vi "Build Chart Update.vi"(4 "error in (no error)":errorcluster, 7 "State Machine Data":T2) -> (0 "error out":errorcluster, 3 "Chart Sample":T1)   [LabVIEW 2015, in "Startup Processes.lvlib"]
uses:
  Startup Processes.lvlib
  _typedefs/State Machine Conditions.ctl
  _typedefs/Machine Modes.ctl
  _typedefs/Subpanel Names.ctl
  Config Data/Config Data.lvclass
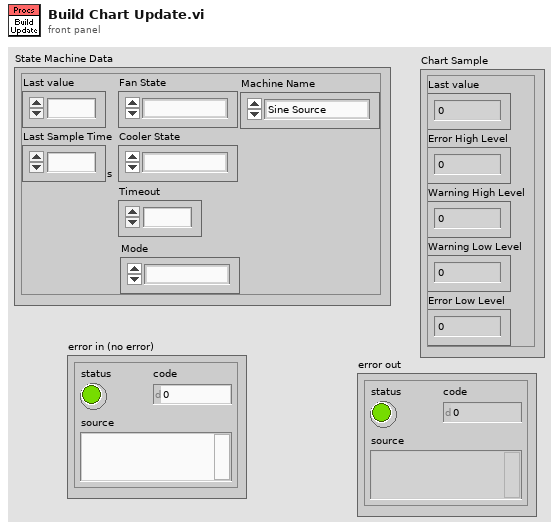
[diagram p1: front panel]
types:
  T1 = cluster{"Last value":dbl, "Error High Level":dbl, "Warning High Level":dbl, "Warning Low Level":dbl, "Error Low Level":dbl}
  T2 = typedef "Startup Processes.lvlib/State Machine Conditions.ctl" = cluster{"Last value":dbl, "Last Sample Time":dbl[unit], "Fan State":enum16{"Off", "On"}, "Cooler State":enum16{"Off", "On"}, "Timeout":i32, "Mode":T3, "Machine Name":T4}
  T3 = typedef "Startup Processes.lvlib/Machine Modes.ctl" = enum16{"Startup", "Run"}
  T4 = typedef "Startup Processes.lvlib/Subpanel Names.ctl" = enum16{"Sine Source", "Ramp Source", "Hen House TC", "Dog House TC", "Out House TC"}
  T5 = cluster{"Error High Level":dbl, "Warning High Level":dbl, "Warning Low Level":dbl, "Error Low Level":dbl, "Sample Interval":dbl[unit]}
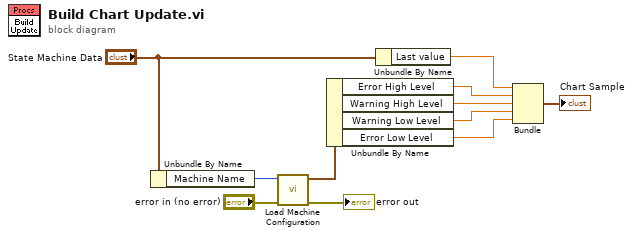
[diagram p0: block diagram]
diagram:
  n1 = Unbundle By Name("State Machine Data") -> ("Machine Name"=w10:T4)
  n2 = call "Load Machine Configuration.vi"("error in (no error)"="error in (no error)", "Instance Name"=w10) -> ("error out"=→"error out":errorcluster, "TC Parameters"=w9:T5)  [unwired: 4 in]
  n3 = Unbundle By Name(w9) -> ("Error High Level"=w8:dbl, "Warning High Level"=w7:dbl, "Warning Low Level"=w6:dbl, "Error Low Level"=w5:dbl)
  n4 = Unbundle By Name("State Machine Data") -> ("Last value"=w4:dbl)
  n5 = Bundle("Last value"=w4, "Error High Level"=w8, "Warning High Level"=w7, "Warning Low Level"=w6, "Error Low Level"=w5) -> (→"Chart Sample":T1)  [unwired: 1 in]
